vi "Global-test.vi"() -> ()   [LabVIEW 2020]
panel:
  in  "File":string
  out "Boolean":bool
  in  "String":string
  in  "Test":dbl
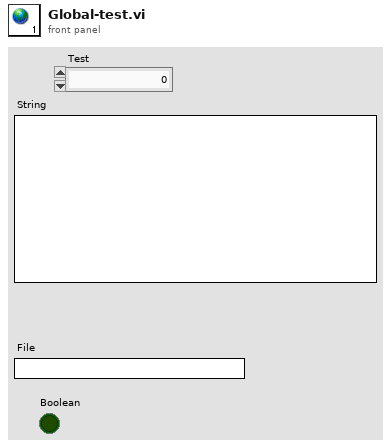
[diagram p1: front panel]
diagram:
